vi "tsc--RGB to Color.vi"(9 "B":u8, 10 "G":u8, 11 "R":u8) -> (3 "Color":u32(colorbox))   [LabVIEW 2021, in "Material SubVIs.lvlib"]
doc: "Re-entrant capable version of RGB to Color.vi.\n\nSimply provides a direct implementation of the subVI contents.\n\n<b>Code Developed By:</b> +\nDaniel Coons +\nTechnology Service Corporation +\nwww.tsc.com/atcs"
uses:
  Material SubVIs.lvlib
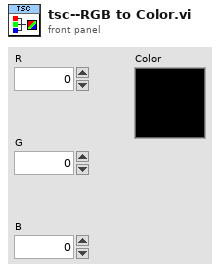
[diagram p1: front panel]
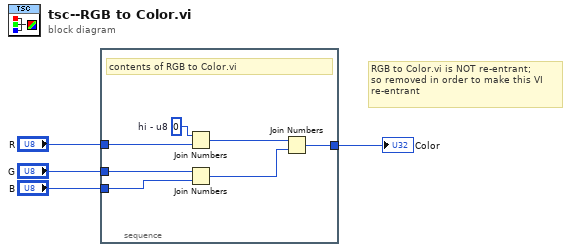
[diagram p0: block diagram]
diagram:
  # "RGB to Color.vi is NOT re-entrant;\nso removed in order to make this VI \nre-entrant"
  n1 = stacked-sequence {
    tunnel: [w11] -> w1
    tunnel: "B" -> [w8]
    tunnel: "G" -> [w7]
    tunnel: "R" -> [w6]
    frame #0 {
      w5 = u8 0  # hi - u8
      # "contents of RGB to Color.vi"
      n2 = Join Numbers(hi=w5, lo=w6) -> ((hi.lo)=w9:u16)
      n3 = Join Numbers(hi=w7, lo=w8) -> ((hi.lo)=w10:u16)
      n4 = Join Numbers(hi=w9, lo=w10) -> ((hi.lo)=w11:u32)
    }
  }
  "Color" <- w1
